vi "update spot.vi"(7 "dt":dbl=0.2, 10 "kalman result":T2, 11 "Spots":T1(array[cluster])=[{"pos"=[{"weighted sum"=0.0, "n measurements"=0.0, "t values"=[], "x values"=[], "t start"=0.0}, {"weighted sum"=0.0, "n measurements"=0.0, "t values"=[], "x values"=[], "t start"=0.0}, {"weighted sum"=0.0, "n measurements"=0.0, "t values"=[], "x values"=[], "t start"=0.0}], "red"={"weighted sum"=0.0, "n measurements"=0.0, "t values"=[], "x values"=[], "t start"=0.0}, "green"={"weighted sum"=0.0, "n measurements"=0.0, "t values"=[], "x values"=[], "t start"=0.0}, "ratio"={"weighted sum"=0.0, "n measurements"=0.0, "t values"=[], "x values"=[], "t start"=0.0}, "SPPF state"={"theta"=[], "w"=[], "elapsed time"=0.0}}]) -> (3 "spots out":T1(array[cluster]))   [LabVIEW 2010]
uses:
  kalman_result_scaled.ctl
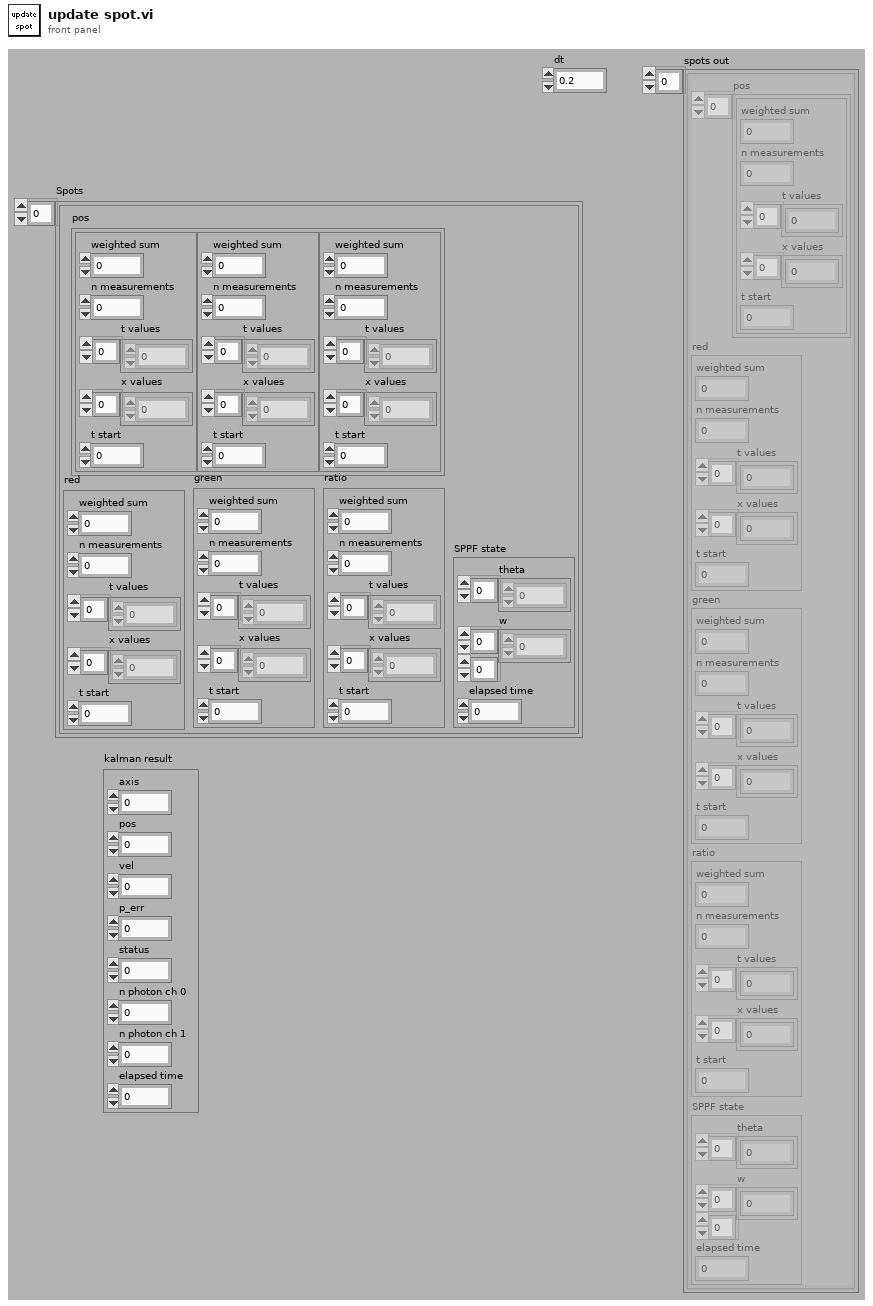
[diagram p1: front panel]
types:
  T1 = cluster{"pos":cluster{"weighted sum":dbl, "n measurements":dbl, "t values":dbl[], "x values":dbl[], "t start":dbl}[], "red":cluster{"weighted sum":dbl, "n measurements":dbl, "t values":dbl[], "x values":dbl[], "t start":dbl}, "green":cluster{"weighted sum":dbl, "n measurements":dbl, "t values":dbl[], "x values":dbl[], "t start":dbl}, "ratio":cluster{"weighted sum":dbl, "n measurements":dbl, "t values":dbl[], "x values":dbl[], "t start":dbl}, "SPPF state":cluster{"theta":dbl[], "w":dbl[][], "elapsed time":dbl}}[]
  T2 = typedef "kalman_result_scaled.ctl" = cluster{"axis":u8, "pos":dbl, "vel":dbl, "p_err":dbl, "status":u32, "n photon ch 0":u32, "n photon ch 1":u32, "elapsed time":dbl}
  T3 = cluster{"pos":cluster{"weighted sum":dbl, "n measurements":dbl, "t values":dbl[], "x values":dbl[], "t start":dbl}[], "red":cluster{"weighted sum":dbl, "n measurements":dbl, "t values":dbl[], "x values":dbl[], "t start":dbl}, "green":cluster{"weighted sum":dbl, "n measurements":dbl, "t values":dbl[], "x values":dbl[], "t start":dbl}, "ratio":cluster{"weighted sum":dbl, "n measurements":dbl, "t values":dbl[], "x values":dbl[], "t start":dbl}, "SPPF state":cluster{"theta":dbl[], "w":dbl[][], "elapsed time":dbl}}
  T4 = cluster{"theta":dbl[], "w":dbl[][], "elapsed time":dbl}
  T5 = cluster{"weighted sum":dbl, "n measurements":dbl, "t values":dbl[], "x values":dbl[], "t start":dbl}
  T6 = cluster{"weighted sum":dbl, "n measurements":dbl, "t values":dbl[], "x values":dbl[], "t start":dbl}[]
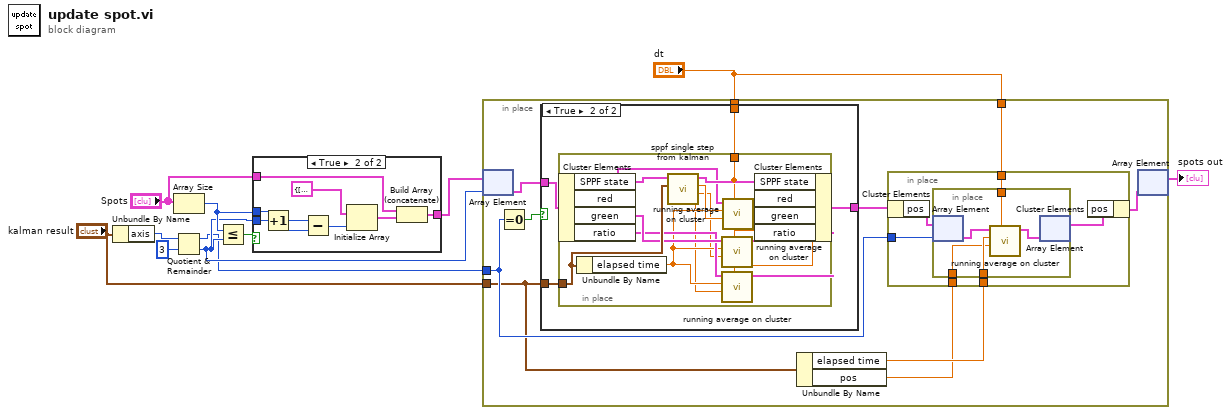
[diagram p0: block diagram]
diagram:
  n1 = Unbundle By Name("kalman result") -> ("axis"=w11:u8)
  n2 = Array Size(array="Spots") -> (size(s)=w8:i32)
  n3 = Quotient & Remainder(x=w11, y=u8 3) -> (x-y*floor(x/y)=w1:u8, floor(x/y)=w2:u8)
  n4 = Less Or Equal?(x=w8, y=w2) -> (x <= y?=w9:bool)
  n5 = case shown="True" w9 {
    tunnel: w2 -> [_ w20]
    tunnel: w8 -> [_ w19]
    tunnel: "Spots" -> [w12 w14]
    tunnel: [w12 w13] -> w6
    frame False {
    }
    frame True {
      n6 = Increment(x=w20) -> (x+1=w18:u8)
      n7 = Subtract(x=w18, y=w19) -> (x-y=w16:i32)
      n8 = Initialize Array(T3 {"pos"=[{"weighted sum"=0.0, "n measurements"=0.0, "t values"=[], "x values"=[], "t start"=0.0}, {"weighted sum"=0.0, "n measurements"=0.0, "t values"=[], "x values"=[], "t start"=0.0}, {"weighted sum"=0.0, "n measurements"=0.0, "t values"=[], "x values"=[], "t start"=0.0}], "red"={"weighted sum"=0.0, "n measurements"=0.0, "t values"=[], "x values"=[], "t start"=0.0}, "green"={"weighted sum"=0.0, "n measurements"=0.0, "t values"=[], "x values"=[], "t start"=0.0}, "ratio"={"weighted sum"=0.0, "n measurements"=0.0, "t values"=[], "x values"=[], "t start"=0.0}, "SPPF state"={"theta"=[], "w"=[], "elapsed time"=0.0}} ("spot"), w16) -> (w15:T1)
      n9 = Build Array (concatenate)(w14, w15) -> (w13:T1)
    }
  }
  n10 = in-place {
    in-place-border: w1 -> [w27]
    in-place-border: "kalman result" -> [w26]
    in-place-border: "dt" -> [w22]
    in-place-border: "dt" -> [w21]
    n11 = in-place-array #1(w6, w2) -> (w30:T3)
    n12 = Equal To 0?(x=w27) -> (x = 0?=w29:bool)
    n13 = case shown="True" w29 {
      tunnel: w30 -> [w42 w46]
      tunnel: w26 -> [_ w45]
      tunnel: [w42 w44] -> w28
      tunnel: w22 -> [_ w43]
      frame False {
      }
      frame True {
        n14 = in-place {
          in-place-border: w45 -> [w58]
          in-place-border: w43 -> [w47]
          n15 = in-place-cluster #2(w46) -> ("SPPF state"=w60:T4, "red"=w56:T5, "green"=w55:T5, "ratio"=w54:T5)
          n16 = Unbundle By Name(w58) -> ("elapsed time"=w53:dbl)
          n17 = call "sppf single step from kalman.vi"("kalman result"=w58, "SPPF state"=w60) -> ("ratio"=w51:dbl, "green rate"=w52:dbl, "red rate"=w57:dbl, "SPPF state out"=w59:T4)  [unwired: 5 in, 1 out]
          n18 = call "running average on cluster.vi"("dt"=w47, "x"=w52, "t"=w53, "averaging state cluster"=w55) -> ("averaging state cluster out"=w49:T5)  [unwired: 7 in]
          n19 = call "running average on cluster.vi"("dt"=w47, "x"=w51, "t"=w53, "averaging state cluster"=w54) -> ("averaging state cluster out"=w48:T5)  [unwired: 7 in]
          n20 = call "running average on cluster.vi"("dt"=w47, "x"=w57, "t"=w53, "averaging state cluster"=w56) -> ("averaging state cluster out"=w50:T5)  [unwired: 7 in]
          n21 = in-place-cluster #2("SPPF state"=w59, "red"=w50, "green"=w49, "ratio"=w48) -> (w44:T3)
        }
      }
    }
    n22 = Unbundle By Name(w26) -> ("elapsed time"=w25:dbl, "pos"=w24:dbl)
    n23 = in-place {
      in-place-border: w27 -> [w35]
      in-place-border: w25 -> [w34]
      in-place-border: w24 -> [w33]
      in-place-border: w21 -> [w31]
      n24 = in-place-cluster #3(w28) -> ("pos"=w36:T6)
      n25 = in-place {
        in-place-border: w34 -> [w40]
        in-place-border: w33 -> [w39]
        in-place-border: w31 -> [w37]
        n26 = in-place-array #4(w36, w35) -> (w41:T5)
        n27 = call "running average on cluster.vi"("dt"=w37, "x"=w39, "t"=w40, "averaging state cluster"=w41) -> ("averaging state cluster out"=w38:T5)  [unwired: 7 in]
        n28 = in-place-array #4(w38) -> (w32:T6)  [unwired: 1 out]
      }
      n29 = in-place-cluster #3("pos"=w32) -> (w23:T3)
    }
    n30 = in-place-array #1(w23) -> (→"spots out":T1)  [unwired: 1 out]
  }
